vi "G#Object_GetClassType.vi"(1 "class path":path, 5 "error in (no error)":errorcluster) -> (14 "reference out":refnum<class "G#Object.lvclass">, 19 "error out":errorcluster)   [LabVIEW 2017, in "G#Object.lvclass"]
doc: "Returns an invalid G#Object of the type specified by the class path. Use this VI to dynamically select class type and load it into memory."
uses:
  G#Object.lvclass
  <vilib>/Utility/error.llb/Error Cluster From Error Code.vi
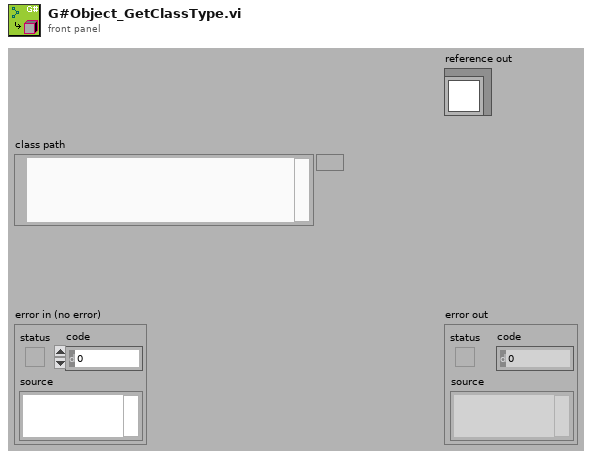
[diagram p1: front panel]
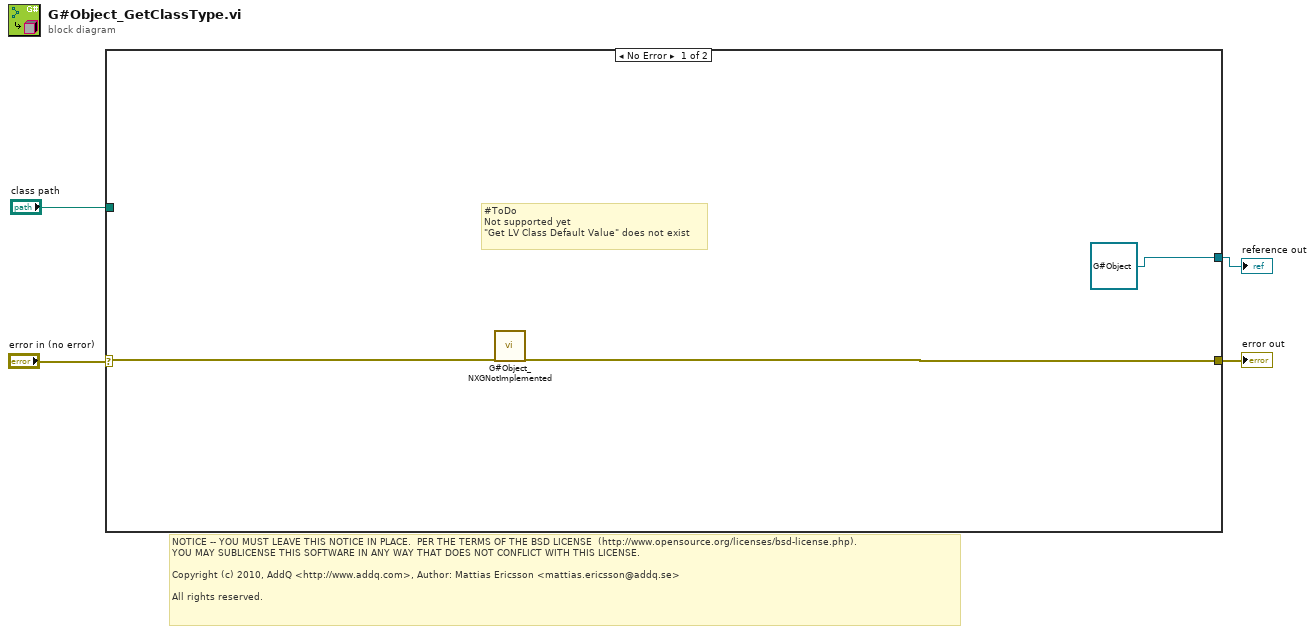
[diagram p0: block diagram]
diagram:
  # "NOTICE -- YOU MUST LEAVE THIS NOTICE IN PLACE.  PER THE TERMS OF THE BSD LICENSE  (http://www.opensource.org/licenses/bsd-license.php).\nYOU MAY SUBLICENSE THIS SOFTWARE IN ANY WAY THAT DOES NOT CONFLICT WITH THIS LICENSE.\n\nCopyright (c) 2010, AddQ <http://www.addq.com>, Author: Mattias Ericsson <mattias.ericsson@addq.se>\n\nAll rights reserved."
  n1 = case shown="No Error" "error in (no error)" {
    selector: "error in (no error)" -> [w6 w8]
    tunnel: [w5 w8] -> w3
    tunnel: "class path" -> [_ _]
    tunnel: [refnum<class "G#Object.lvclass"> refnum ("reference out") _] -> w1
    frame No Error {
      # "#ToDo \nNot supported yet\n\"Get LV Class Default Value\" does not exist"
      n2 = call "G#Object_NXGNotImplemented.vi"("error in"=w6) -> ("error out"=w5:errorcluster)  [unwired: 18 in]
    }
    frame Error {
    }
  }
  "error out" <- w3
  "reference out" <- w1
